vi "BiTest.vi"() -> ()   [LabVIEW 2019]
panel:
  out "XY Graph":cluster{dbl[], i16[]}[](graph)
  in  "Boolean":bool
  in  "AI Count(uSec)":u32=5
  out "Stop":bool
  in  "TE_Segments":i16[](array[numeric])=[0, 0, 0]
  in  "BE_Segments":i16[](array[numeric])=[0, 0, 0]
  in  "RE_Segments":i16[](array[numeric])=[0, 0, 0]
  in  "Segment_uSec":sgl[](array[numeric])=[0.0, 0.0, 0.0]
  in  "BE_Start":i16
  in  "TE_Start":i16
  in  "RE_Start":i16
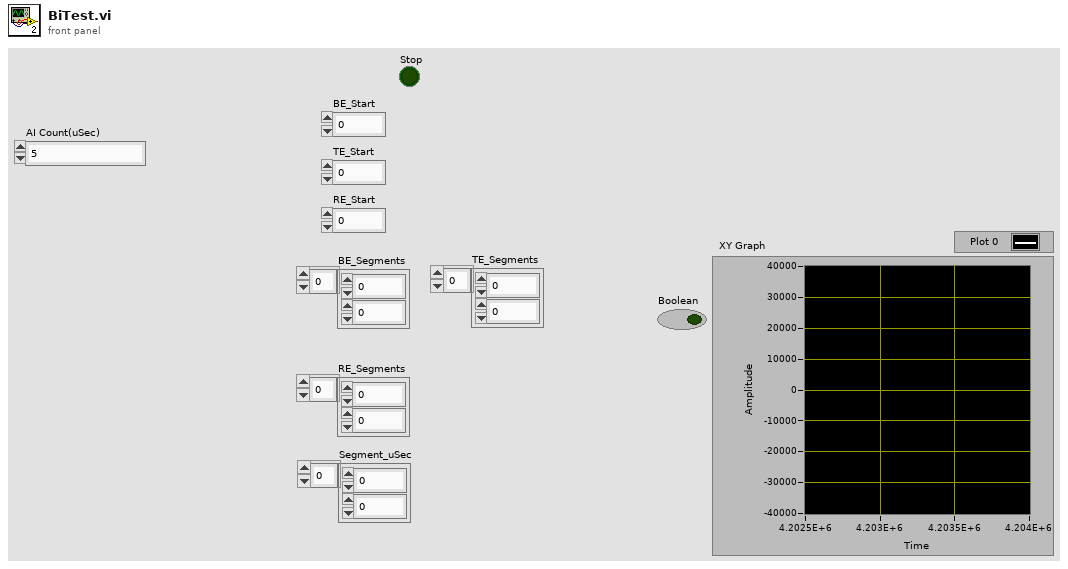
[diagram p1: front panel]
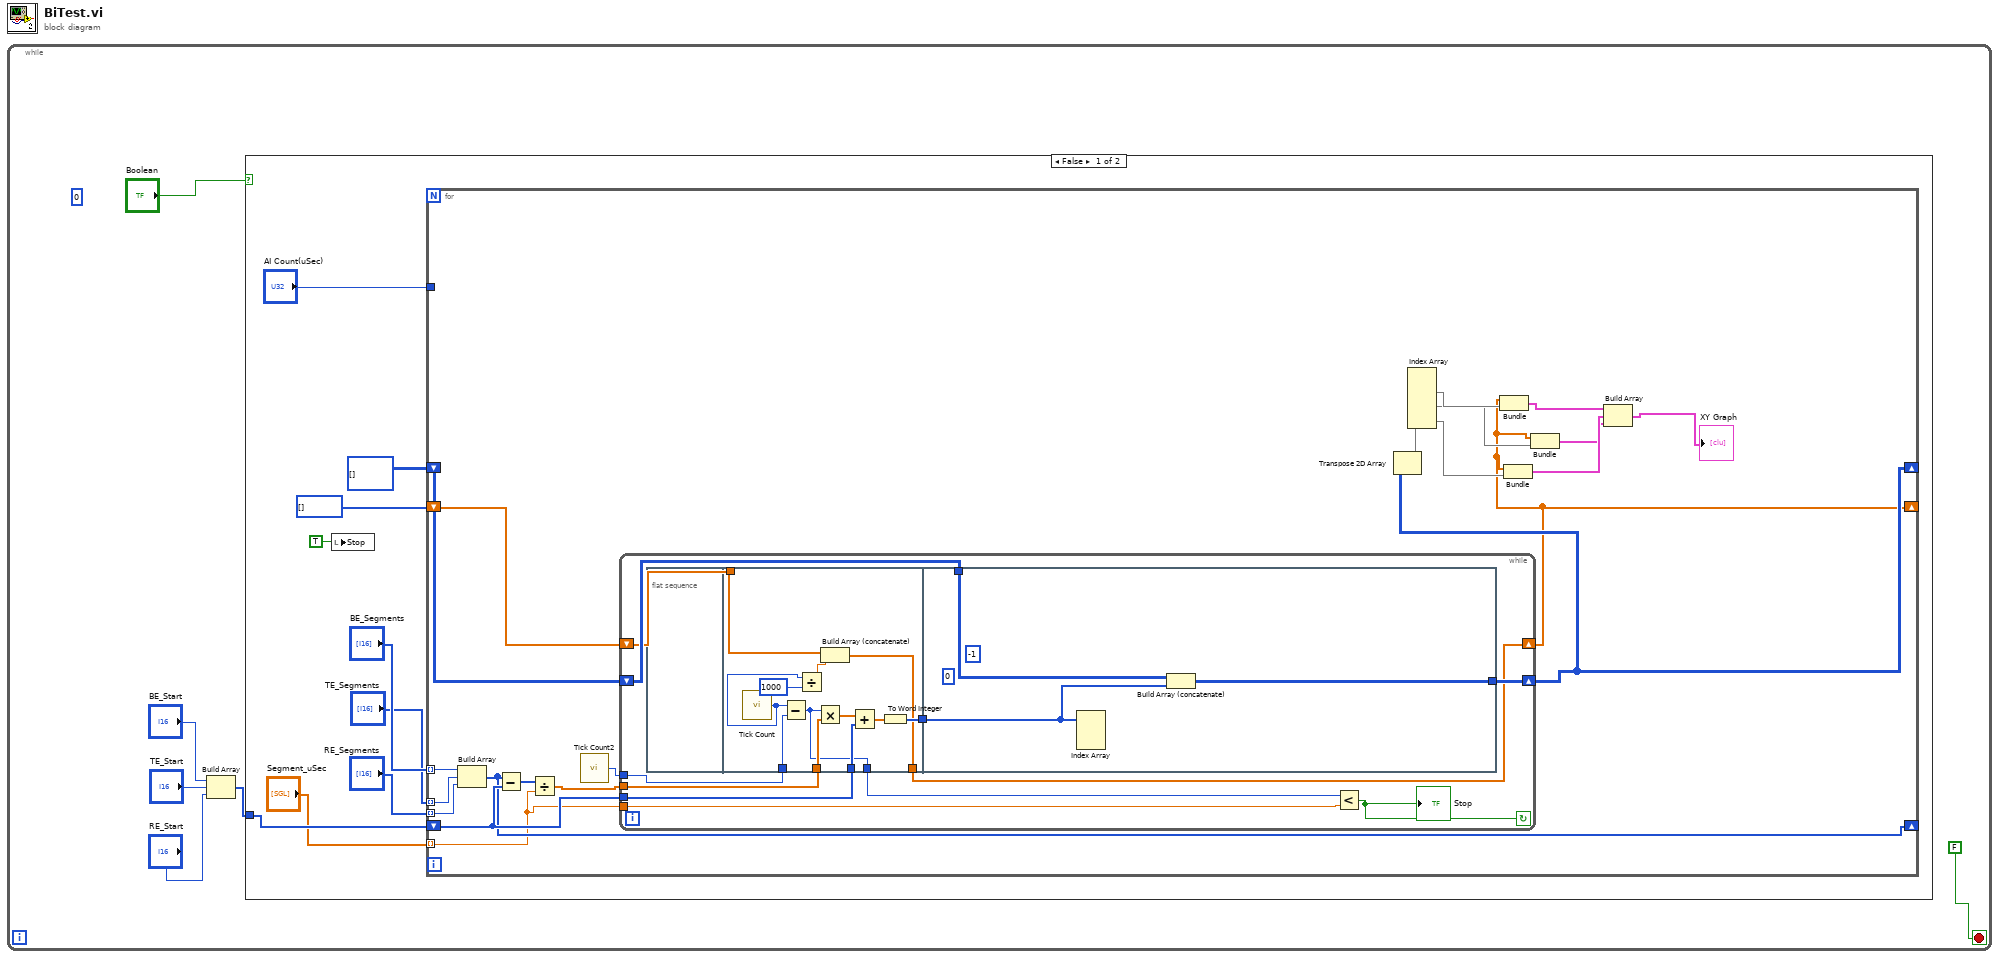
[diagram p0: block diagram]
diagram:
  n1 = while {
    stop <- FALSE stop-if-true
    (unwired) 0 ("Timeout")
    n2 = Build Array("BE_Start", "TE_Start", "RE_Start") -> (w2:i16[])
    n3 = case shown="False" "Boolean" {
      tunnel: w2 -> [w14 _]
      frame False {
        n4 = local write "Stop"(TRUE ("Stop")) -> ()
        n5 = for {
          tunnel: "AI Count(uSec)" -> [_]
          shift-right: [w30] -> _
          shift-left: w14 -> [w31]
          tunnel: "Segment_uSec" -> [w28] mode=indexing
          tunnel: "BE_Segments" -> [w35] mode=indexing
          tunnel: "TE_Segments" -> [w34] mode=indexing
          tunnel: "RE_Segments" -> [w33] mode=indexing
          shift-right: [w25] -> _
          shift-left: i16[][] [] -> [w27]
          shift-right: [w20] -> _
          shift-left: u32[] [] -> [w26]
          n6 = Build Array(w35, w34, w33) -> (w30:i16[])
          n7 = Subtract(x=w30, y=w31) -> (x-y=w32:i16[])
          n8 = Divide(x=w32, y=w28) -> (x/y=w29:sgl[])
          n9 = call "Tick Count2"() -> ("Tick Count(uSec)"=w36:u32)
          n10 = while {
            tunnel: w36 -> [w47]
            tunnel: w31 -> [w46]
            tunnel: w29 -> [w44]
            tunnel: w28 -> [w42]
            shift-right: [w40] -> w25
            shift-left: w27 -> [w39]
            shift-right: [w38] -> w20
            shift-left: w26 -> [w37]
            stop <- w41 continue-if-true
            n11 = flat-sequence {
              tunnel: w47 -> [w59]
              tunnel: w44 -> [w58]
              tunnel: w46 -> [w56]
              tunnel: [w54] -> w45
              tunnel: [w50] -> w43
              tunnel: [w53] -> w38
              tunnel: w37 -> [w52]
              tunnel: w45 -> [w62]
              tunnel: [w61] -> w40
              tunnel: w39 -> [w60]
              frame #0 {
              }
              frame #1 {
                n12 = call "Tick Count"() -> ("Tick Count(uSec)"=w48:u32)
                n13 = Subtract(x=w48, y=w59) -> (x-y=w50:u32)
                n14 = Divide(x=w48, y=u32 1000) -> (x/y=w51:dbl)
                n15 = Multiply(x=w50, y=w58) -> (x*y=w57:sgl[])
                n16 = Build Array (concatenate)(w52, w51) -> (w53:dbl[])
                n17 = Add(x=w57, y=w56) -> (x+y=w55:sgl[])
                n18 = To Word Integer(number=w55) -> (16bit integer=w54:i16[])
              }
              frame #2 {
                (unwired) 0 ("Timeout")
                (unwired) i16 -1 ("Element")
                n19 = Index Array(array=w62) -> ()  [unwired: 3 in, 3 out]
                n20 = Build Array (concatenate)(w60, w62) -> (w61:i16[][])
              }
            }
            n21 = Less?(x=w43, y=w42) -> (x < y?=w41:bool)
            "Stop" <- w41
          }
          n22 = Transpose 2D Array(2D array=w25) -> (transposed array=w16:i16[][])
          n23 = Index Array(array=w16) -> (element #1=w24:i16[], element #2=w22:i16[], element #3=w21:i16[])  [unwired: 6 in]
          n24 = Bundle(w20, w24) -> (w23:cluster{dbl[], i16[]})  [unwired: 1 in]
          n25 = Bundle(w20, w21) -> (w19:cluster{dbl[], i16[]})  [unwired: 1 in]
          n26 = Bundle(w20, w22) -> (w18:cluster{dbl[], i16[]})  [unwired: 1 in]
          n27 = Build Array(w23, w19, w18) -> (→"XY Graph":cluster{dbl[], i16[]}[])
        }
      }
      frame True {
      }
    }
  }
